vi "Get Data Variant.vi"(8 "error in (no error)":errorcluster, 11 "RDMA Plugin Configuration in":refnum<class "RDMA Plugin Configuration.lvclass">) -> (0 "error out":errorcluster, 1 "data version":T1, 2 "data":variant, 3 "RDMA Plugin Configuration out":refnum<class "RDMA Plugin Configuration.lvclass">)   [LabVIEW 2020, in "RDMA.lvlib" / "RDMA Plugin Configuration.lvclass"]
uses:
  RDMA Plugin Configuration.lvclass
  DSF Core.lvlibp/Typedefs/DSF Version Info.ctl
  RDMA Plugin Configuration.lvclass/RDMA Plugin Configuration.ctl
  DSF Core.lvlibp
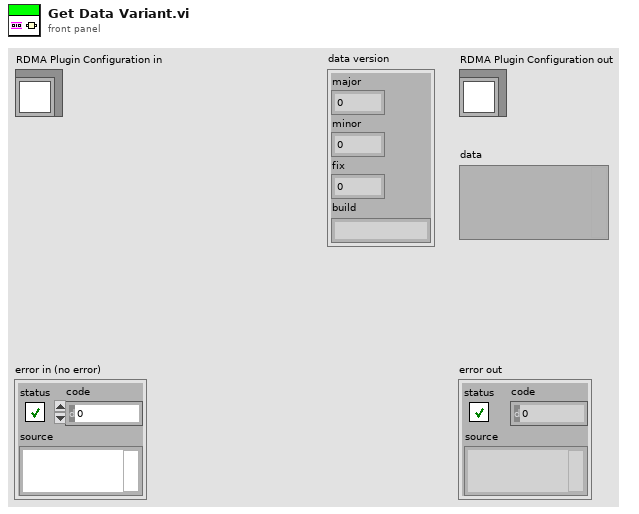
[diagram p1: front panel]
types:
  T1 = typedef "DSF Core.lvlibp/DSF Version Info.ctl" = cluster{"major":u32, "minor":u32, "fix":u32, "build":string}
  T2 = typedef "RDMA.lvlib/RDMA Plugin Configuration.lvclass/Plugin Settings.ctl" = cluster{"initialization timeout s":dbl}
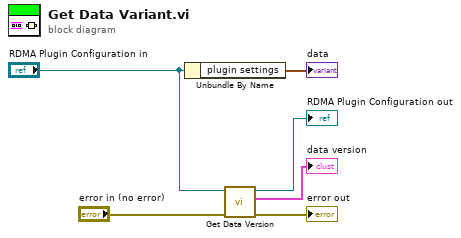
[diagram p0: block diagram]
diagram:
  n1 = Unbundle By Name("RDMA Plugin Configuration in") -> ("plugin settings"=→"data":T2)
  n2 = call-dynamic "Get Data Version.vi"("error in (no error)"="error in (no error)", "RDMA Plugin Configuration in"="RDMA Plugin Configuration in") -> ("error out"=→"error out":errorcluster, "data version"=→"data version":T1, "RDMA Plugin Configuration out"=→"RDMA Plugin Configuration out":refnum<class "RDMA Plugin Configuration.lvclass">)  [unwired: 7 in]
